vi "Global System.vi"() -> ()   [LabVIEW 2017]
uses:
  <vilib>/userdefined/High Color/IMAQdx.ctl
  <vilib>/vision/Pattern Matching.llb/IMAQ Curve Parameters.ctl
  <vilib>/vision/Image Controls.llb/IMAQ Image.ctl
  <vilib>/vision/Measure.llb/Edge Options.ctl
  <vilib>/vision/Measure.llb/Edge Polarity.ctl
  <vilib>/vision/Measure.llb/Straight Edge Options.ctl
  <vilib>/vision/Measure.llb/Straight Edge Process.ctl
  <vilib>/vision/Pattern Matching.llb/IMAQ Match Range Setting.ctl
panel:
  out "码枪结果":bool
  out "CR-CCD1字符定位参数":T4={"Rectangle"={"Left"=0, "Top"=0, "Right"=0, "Bottom"=0, "Rotation"=0.0}, "Settings"={"Curve Parameters"={"Extraction Mode"=0, "Edge Threshold"=35, "Edge Filter Size"=1, "Min Length"=25, "Row Search Step Size"=15, "Col Search Step Size"=15, "Max Endpoint Gap"=10, "Closed"=FALSE, "Subpixel"=FALSE}, "Match Mode"={"Rotation"=TRUE, "Scale"=FALSE, "Occlusion"=TRUE, "Reserved 1"=FALSE, "Reserved 2"=FALSE, "Reserved 3"=FALSE}, "Range Settings"=[{"Match Constraints"=0, "Min"=-17.0, "Max"=17.0}, {"Match Constraints"=2, "Min"=0.0, "Max"=25.0}], "Number of Matches"=1, "Minimum Match Score"=400.0, "SubPixel Accuracy"=FALSE, "Adv. Geometric Match Options 2"=[{"Setup Data Item"=21, "Item Value"=0.0}, {"Setup Data Item"=22, "Item Value"=1.0}]}, "Template File Path"=path "F:/Inspect System -2/Source Code/Template Program/程序1/字符定位模板.png"} {"Settings"."Curve Parameters"."Extraction Mode" items=["Normal", "Uniform Regions"]; "Settings"."Curve Parameters"."Edge Filter Size" items=["Fine", "Normal", "Contour Tracing"]; "Settings"."Curve Parameters"."Max Endpoint Gap" min=0; "Settings"."Curve Parameters"."Col Search Step Size" min=1 max=255 step=1; "Settings"."Curve Parameters"."Row Search Step Size" min=1 max=255 step=1; "Settings"."Curve Parameters"."Min Length" min=0; "Settings"."Curve Parameters"."Edge Threshold" min=1 max=350 step=1; "Settings"."Range Settings"."Max" format="%.2f"; "Settings"."Range Settings"."Min" format="%.2f"; "Settings"."Range Settings"."Match Constraints" items=["Rotation Angle (degrees)", "Scale Factor (%)", "Occlusion (%)"]; "Settings"."Adv. Geometric Match Options 2"."Setup Data Item" items=["Curve Extraction Mode", "Curve Edge Threshold", "Curve Edge Filter Size", "Min Curve Length", "Curve Row Search Step Size", "Curve Col Search Step Size", "Curve Max Endpoint Gap", "Extract Closed Curves", "Enable Subpixel Curve Extraction", "Enable Correlation Score", "Enable Subpixel Accuracy", "Subpixel Iterations", "Subpixel Tolerance", "Initial Match List Length", "Enable Target Template Curve Score", "Min Match Separation Distance", "Min Match Separation Angle", "Min Match Separation Scale", "Max Match Overlap", "Enable Coarse Result", "Enable Calibration Support", "Enable Contrast Reversal", "Search Strategy", "Refinement Match Factor", "Subpixel Match Factor"]; "Rectangle"."Rotation" format="%.2f"; "Rectangle"."Left" scale=0.0..1024.0; "Rectangle"."Right" scale=0.0..1024.0}
  out "扫码次数计数":dbl
  out "CR位置范围设定":T5={"位置1"={"上限"=726.0, "下限"=686.0}, "位置2"={"上限"=874.0, "下限"=834.0}, "位置3"={"上限"=997.0, "下限"=957.0}, "位置4"={"上限"=1139.0, "下限"=1099.0}, "位置5"={"上限"=1283.0, "下限"=1243.0}, "位置6"={"上限"=1429.0, "下限"=1389.0}, "位置7"={"上限"=1576.0, "下限"=1536.0}, "位置8"={"上限"=1728.0, "下限"=1688.0}, "位置9"={"上限"=1879.0, "下限"=1839.0}, "位置10"={"上限"=2036.0, "下限"=1996.0}}
  out "CR- 字符检测参数 2":T6={"Parameters (OCR/OCV 1)"={"Threshold Data"={"Method"=enum."Local", "Looking for"=1, "Color Mode"=0, "Kernel Size"={"Width"=32, "Height"=32}, "Ranges"=[{"Min"=1, "Max"=255}]}, "Reject Border"=TRUE, "Number Of Erosions"=0, "Size & Spacing"={"Segment Algorithm"=0, "Min Bounding Rect Width"=1, "Max Bounding Rect Width"=65536, "Min Bounding Rect Height"=1, "Max Bounding Rect Height"=65536, "Min Character Size"=20, "Max Character Size"=65536, "Min Char Spacing"=1, "Max Horiz Element Spacing"=1, "Max Vert Element Spacing"=0, "Max Space Distance"=65536}, "Read Options"={"Read Strategy"=1, "Read Resolution"=2, "Scale Dependant"=FALSE, "Aspect Ratio"=400, "Acceptance Level"=700, "Substitution Character"="?", "MultiLine"=TRUE}, "Valid Characters"=[], "Use Text Pattern"=FALSE, "Orientation"=0, "# Lines Expected"=0, "Number of Blocks"=4}, "Rectangle"={"Left"=0, "Top"=0, "Right"=0, "Bottom"=0, "Rotation"=0.0}, "字符长度判定"=0.0, "Reference System"={"Origin"={"X"=1245.2058, "Y"=1038.7815}, "Angle (deg)"=0.021420227, "Axis Reference"=0}, "File Path (字符库)"=path "D:/Inspect System/Source Code/Template Program/字符模板.abc", "File Path (连接件模板)"=path "D:/Inspect System/Source Code/Template Program/字符检测定位模板.png", "Url"="http://10.6.1.31:8080/MesInnerpackLineIO.asmx", "accessKey"="a45b2d3334ffs_\na45b2d3334ffs_"} {"Reference System"."Axis Reference" items=["Direct", "Indirect"]; "Rectangle"."Rotation" min=-90.0 max=90.0 step=1.0 format="%.2f"; "Rectangle"."Left" scale=0.0..1024.0; "Rectangle"."Right" scale=0.0..1024.0; "Parameters (OCR/OCV 1)"."Threshold Data"."Looking for" items=["Light on Dark", "Dark on Light"]; "Parameters (OCR/OCV 1)"."Threshold Data"."Color Mode" items=["RGB", "HSL", "HSV", "HSI"]; "Parameters (OCR/OCV 1)"."Size & Spacing"."Segment Algorithm" items=["None", "Shortest Segment", "Legacy Auto Split"]; "Parameters (OCR/OCV 1)"."Read Options"."Read Strategy" items=["Aggressive", "Conservative"]; "Parameters (OCR/OCV 1)"."Read Options"."Read Resolution" items=["Low", "Medium", "High"]; "Parameters (OCR/OCV 1)"."Valid Characters"."Pre-defined characters" items=["Any Character", "User-defined Characters", "Alphabetic", "Alphanumeric", "Uppercase Letters", "Lowercase Letters", "Decimal Digits", "Hexadecimal Digits", "Pattern", "Force Space"]; "Parameters (OCR/OCV 1)"."Orientation" items=["Baseline inside", "Baseline outside"]}
  in  "CR- 衬丝检测ROI参数":T8 {"Line 2"."Start X" scale=0.0..1024.0; "Line 2"."End X" scale=0.0..1024.0; "clamp Rectangle"."Rotation" min=-90.0 max=90.0 step=1.0 format="%.2f"; "clamp Rectangle"."Left" scale=0.0..1024.0; "clamp Rectangle"."Right" scale=0.0..1024.0; "Line 1"."Start X" scale=0.0..1024.0; "Line 1"."End X" scale=0.0..1024.0; "find straight edge Rectangle"."Rotation" min=-90.0 max=90.0 step=1.0 format="%.2f"; "find straight edge Rectangle"."Left" scale=0.0..1024.0; "find straight edge Rectangle"."Right" scale=0.0..1024.0}
  in  "衬丝检测基础参数":T9={"IsNorImage"=TRUE, "Exposure Values"=100289, "ImagePath"=path "C:/Users/hedongpo/Desktop/514-hdp/Alignment Assemble System/Test Picture/B/3.bmp"} caption="参数界面" {"Exposure Values" scale=0.0..200000.0}
  out "CR- 衬丝检测参数":T12={"Settings (Clamp (Rake) 1)"={"Contrast"=154, "Filter width"=4, "Steepness"=2, "Subsampling Ratio"=5, "Show Search Area"=TRUE, "Show Search Lines"=TRUE, "Show Edges Found"=TRUE, "Show Result"=TRUE}, "Options (Find Straight Edge 1)"={"Search Direction"=0, "Edge Options"={"Edge Polarity"=0, "Kernel Size"=3, "Width"=1, "Minimum Edge Strength"=65.0, "Interpolation Type"=enum."Bilinear Fixed", "Data Processing Method"=enum."Average"}, "Show Search Area"=TRUE, "Show Search Lines"=TRUE, "Show Edges Found"=TRUE, "Show Result"=TRUE, "Search Area Color"=65280, "Search Lines Color"=255, "Edge Locations Color"=16776960, "Result Color"=16711680, "Overlay Group Name"=""}, "相对距离设定"={"上限"=0.0, "下限"=0.0}, "衬丝直径设定"={"上限"=0.0, "下限"=0.0}, "保护套直径设定"={"上限"=0.0, "下限"=0.0}, "Edge Options (Edge Detector 1)"={"Edge Polarity"=0, "Kernel Size"=3, "Width"=3, "Minimum Edge Strength"=10.0, "Interpolation Type"=enum."Bilinear Fixed", "Data Processing Method"=enum."Average"}, "保护套标准位置"={"Start X"=0, "Start Y"=0, "End X"=0, "End Y"=0}} {"保护套标准位置"."Start X" scale=0.0..1024.0; "保护套标准位置"."End X" scale=0.0..1024.0; "Edge Options (Edge Detector 1)"."Edge Polarity" items=["All Edges", "Rising Edges", "Falling Edges"]; "Options (Find Straight Edge 1)"."Search Direction" items=["Left to Right", "Right to Left", "Top to Bottom", "Bottom to Top"]; "Options (Find Straight Edge 1)"."Edge Options"."Edge Polarity" items=["All Edges", "Rising Edges", "Falling Edges"]; "Options (Find Straight Edge 1)"."Edge Options"."Minimum Edge Strength" format="%.2f"; "Options (Find Straight Edge 1)"."Edge Options"."Width" step=2; "Options (Find Straight Edge 1)"."Edge Options"."Kernel Size" step=2}
  out "颗粒物检测1基础参数 2":T14={"IsNorImage"=TRUE, "Exposure Values"=100289, "ImagePath"=path "C:/Users/hedongpo/Desktop/514-hdp/Alignment Assemble System/Test Picture/B/3.bmp", "相机选择"="cam4"} caption="参数界面" {"Exposure Values" scale=0.0..200000.0}
  in  "字符检测基础参数":T9={"IsNorImage"=TRUE, "Exposure Values"=100289, "ImagePath"=path "C:/Users/hedongpo/Desktop/514-hdp/Alignment Assemble System/Test Picture/B/3.bmp"} caption="参数界面" {"Exposure Values" scale=0.0..200000.0}
  in  "扫码枪基础参数":T15 caption="参数界面"
  in  "CR导丝纤维毛发检测3参数":T16={"Curve Extraction Settings "={"Extraction Mode"=0, "Edge Threshold"=25, "Edge Filter Size"=1, "Min Length"=19, "Row Search Step Size"=5, "Col Search Step Size"=5, "Max Endpoint Gap"=10, "Closed"=FALSE, "Subpixel"=FALSE}, "Color Mode (Histogram 1)"=0, "Range (Threshold 1)"={"Lower value"=62.0, "Upper value"=255.0}, "Clamp Settings (Max Clamp 1)"={"Angle Range (+/-)"=10.0, "Edge Polarity"={"Start"=0, "End"=0}}, "Settings (Clamp (Rake) 1)"={"Contrast"=6, "Filter width"=5, "Steepness"=2, "Subsampling Ratio"=5, "Show Search Area"=TRUE, "Show Search Lines"=TRUE, "Show Edges Found"=TRUE, "Show Result"=TRUE}, "直径设定"={"Lower value"=62.0, "Upper value"=255.0}} {"Clamp Settings (Max Clamp 1)"."Edge Polarity"."Start" items=["Any", "Rising", "Falling"]; "Clamp Settings (Max Clamp 1)"."Edge Polarity"."End" items=["Any", "Rising", "Falling"]; "Color Mode (Histogram 1)" items=["RGB", "HSL", "HSV", "HSI"]; "Curve Extraction Settings"."Extraction Mode" items=["Normal", "Uniform Regions"]; "Curve Extraction Settings"."Edge Filter Size" items=["Fine", "Normal", "Contour Tracing"]; "Curve Extraction Settings"."Max Endpoint Gap" min=0; "Curve Extraction Settings"."Col Search Step Size" min=1 max=255 step=1; "Curve Extraction Settings"."Row Search Step Size" min=1 max=255 step=1; "Curve Extraction Settings"."Min Length" min=0; "Curve Extraction Settings"."Edge Threshold" min=1 max=350 step=1}
  in  "CR颗粒物检测3参数":T17={"Rectangle"={"Left"=0, "Top"=0, "Right"=0, "Bottom"=0, "Rotation"=0.0}, "Threshold Limits (Threshold 1)"={"Lower value"=6.0, "Upper value"=245.0}, "Keep/Remove Particles "=FALSE, "Connectivity 4/8 (8) "=TRUE, "Selection Values (Particle Filter 1)"=[{"Measurement Parameter"=35, "Range Lower Value"=80.0, "Range Upper Value"=16332.0, "Range"=FALSE, "Measurement Type"=FALSE}], "Corner Options (Feature Detection 1)"={"Detector type"=enum."Harris Corner", "Kernel size"=7, "Min Corner Point Strength"=32.0}, "Pyramid level (Feature Detection 1)"=3, "Method "=2, "Look For"=0, "Method 2"=2, "ROI Descriptor (Clamp (Rake) 1)"={"Global Rectangle"=[162, 394, 420, 1807], "Contours"=[{"ID"=enum."External", "Type"=12, "Coordinates"=[162, 394, 420, 1807, 0]}]}} {"Method" items=["clustering", "entropy", "metric", "moments", "inter-class variance"]; "Look For" items=["Bright Objects", "Dark Objects"]; "Method 2" items=["clustering", "entropy", "metric", "moments", "inter-class variance"]; "ROI Descriptor (Clamp (Rake) 1)"."Contours"."Type" items=["No Selection", "Point", "Line", "Rectangle", "Oval", "Polygon", "Freehand Region", "Annulus", "Unused2", "Unused3", "Broken Line", "Freehand Line", "Rotated Rectangle"]; "Selection Values (Particle Filter 1)"."Measurement Parameter" items=["Center of Mass X", "Center of Mass Y", "First Pixel X", "First Pixel Y", "Bounding Rect Left", "Bounding Rect Top", "Bounding Rect Right", "Bounding Rect Bottom", "Max Feret Diameter Start X", "Max Feret Diameter Start Y", "Max Feret Diameter End X", "Max Feret Diameter End Y", "Max Horiz. Segment Length Left", "Max Horiz. Segment Length Right", "Max Horiz. Segment Length Row", "-", "Bounding Rect Width", "Bounding Rect Height", "Bounding Rect Diagonal", "Perimeter", "Convex Hull Perimeter", "Holes' Perimeter", "Max Feret Diameter", "Equivalent Ellipse Major Axis", "Equivalent Ellipse Minor Axis", "Equivalent Ellipse Minor Axis (Feret)", "Equivalent Rect Long Side", "Equivalent Rect Short Side", "Equivalent Rect Diagonal", "Equivalent Rect Short Side (Feret)", "Average Horiz. Segment Length", "Average Vert. Segment Length", "Hydraulic Radius", "Waddel Disk Diameter", "-", "Area", "Holes' Area", "Particle & Holes' Area", "Convex Hull Area", "Image Area", "-", "Number of Holes", "Number of Horiz. Segments", "Number of Vert. Segments", "-", "Orientation", "Max Feret Diameter Orientation", "-", "% Area/Image Area", "% Area/(Particle & Holes' Area)", "Ratio of Equivalent Ellipse Axes", "Ratio of Equivalent Rect Sides", "-", "Elongation Factor", "Compactness Factor", "Heywood Circularity Factor", "Type Factor", "-", "Sum X", "Sum Y", "Sum XX", "Sum XY", "Sum YY", "Sum XXX", "Sum XXY", "Sum XYY", "Sum YYY", "-", "Moment of Inertia XX", "Moment of Inertia XY", "Moment of Inertia YY", "Moment of Inertia XXX", "Moment of Inertia XXY", "Moment of Inertia XYY", "Moment of Inertia YYY", "Norm. Moment of Inertia XX", "Norm. Moment of Inertia XY", "Norm. Moment of Inertia YY", "Norm. Moment of Inertia XXX", "Norm. Moment of Inertia XXY", "Norm. Moment of Inertia XYY", "Norm. Moment of Inertia YYY", "Hu Moment 1", "Hu Moment 2", "Hu Moment 3", "Hu Moment 4", "Hu Moment 5", "Hu Moment 6", "Hu Moment 7"]; "Rectangle"."Rotation" min=-90.0 max=90.0 step=1.0 format="%.2f"; "Rectangle"."Left" scale=0.0..1024.0; "Rectangle"."Right" scale=0.0..1024.0}
  in  "CR颗粒物检测2参数":T17={"Rectangle"={"Left"=0, "Top"=0, "Right"=0, "Bottom"=0, "Rotation"=0.0}, "Threshold Limits (Threshold 1)"={"Lower value"=6.0, "Upper value"=245.0}, "Keep/Remove Particles "=FALSE, "Connectivity 4/8 (8) "=TRUE, "Selection Values (Particle Filter 1)"=[{"Measurement Parameter"=35, "Range Lower Value"=80.0, "Range Upper Value"=16332.0, "Range"=FALSE, "Measurement Type"=FALSE}], "Corner Options (Feature Detection 1)"={"Detector type"=enum."Harris Corner", "Kernel size"=7, "Min Corner Point Strength"=32.0}, "Pyramid level (Feature Detection 1)"=3, "Method "=2, "Look For"=0, "Method 2"=2, "ROI Descriptor (Clamp (Rake) 1)"={"Global Rectangle"=[162, 394, 420, 1807], "Contours"=[{"ID"=enum."External", "Type"=12, "Coordinates"=[162, 394, 420, 1807, 0]}]}} {"Method" items=["clustering", "entropy", "metric", "moments", "inter-class variance"]; "Look For" items=["Bright Objects", "Dark Objects"]; "Method 2" items=["clustering", "entropy", "metric", "moments", "inter-class variance"]; "ROI Descriptor (Clamp (Rake) 1)"."Contours"."Type" items=["No Selection", "Point", "Line", "Rectangle", "Oval", "Polygon", "Freehand Region", "Annulus", "Unused2", "Unused3", "Broken Line", "Freehand Line", "Rotated Rectangle"]; "Selection Values (Particle Filter 1)"."Measurement Parameter" items=["Center of Mass X", "Center of Mass Y", "First Pixel X", "First Pixel Y", "Bounding Rect Left", "Bounding Rect Top", "Bounding Rect Right", "Bounding Rect Bottom", "Max Feret Diameter Start X", "Max Feret Diameter Start Y", "Max Feret Diameter End X", "Max Feret Diameter End Y", "Max Horiz. Segment Length Left", "Max Horiz. Segment Length Right", "Max Horiz. Segment Length Row", "-", "Bounding Rect Width", "Bounding Rect Height", "Bounding Rect Diagonal", "Perimeter", "Convex Hull Perimeter", "Holes' Perimeter", "Max Feret Diameter", "Equivalent Ellipse Major Axis", "Equivalent Ellipse Minor Axis", "Equivalent Ellipse Minor Axis (Feret)", "Equivalent Rect Long Side", "Equivalent Rect Short Side", "Equivalent Rect Diagonal", "Equivalent Rect Short Side (Feret)", "Average Horiz. Segment Length", "Average Vert. Segment Length", "Hydraulic Radius", "Waddel Disk Diameter", "-", "Area", "Holes' Area", "Particle & Holes' Area", "Convex Hull Area", "Image Area", "-", "Number of Holes", "Number of Horiz. Segments", "Number of Vert. Segments", "-", "Orientation", "Max Feret Diameter Orientation", "-", "% Area/Image Area", "% Area/(Particle & Holes' Area)", "Ratio of Equivalent Ellipse Axes", "Ratio of Equivalent Rect Sides", "-", "Elongation Factor", "Compactness Factor", "Heywood Circularity Factor", "Type Factor", "-", "Sum X", "Sum Y", "Sum XX", "Sum XY", "Sum YY", "Sum XXX", "Sum XXY", "Sum XYY", "Sum YYY", "-", "Moment of Inertia XX", "Moment of Inertia XY", "Moment of Inertia YY", "Moment of Inertia XXX", "Moment of Inertia XXY", "Moment of Inertia XYY", "Moment of Inertia YYY", "Norm. Moment of Inertia XX", "Norm. Moment of Inertia XY", "Norm. Moment of Inertia YY", "Norm. Moment of Inertia XXX", "Norm. Moment of Inertia XXY", "Norm. Moment of Inertia XYY", "Norm. Moment of Inertia YYY", "Hu Moment 1", "Hu Moment 2", "Hu Moment 3", "Hu Moment 4", "Hu Moment 5", "Hu Moment 6", "Hu Moment 7"]; "Rectangle"."Rotation" min=-90.0 max=90.0 step=1.0 format="%.2f"; "Rectangle"."Left" scale=0.0..1024.0; "Rectangle"."Right" scale=0.0..1024.0}
  in  "扫码枪参数":T18={"IsNorImage"=TRUE, "Exposure Values"=100289, "ImagePath"=path "C:/Users/hedongpo/Desktop/514-hdp/Alignment Assemble System/Test Picture/B/3.bmp", "数据输出"="", "结果显示"=FALSE} caption="参数界面" {"Exposure Values" scale=0.0..200000.0}
  in  "CR纤维毛发检测1参数":T16={"Curve Extraction Settings "={"Extraction Mode"=0, "Edge Threshold"=25, "Edge Filter Size"=1, "Min Length"=19, "Row Search Step Size"=5, "Col Search Step Size"=5, "Max Endpoint Gap"=10, "Closed"=FALSE, "Subpixel"=FALSE}, "Color Mode (Histogram 1)"=0, "Range (Threshold 1)"={"Lower value"=62.0, "Upper value"=255.0}, "Clamp Settings (Max Clamp 1)"={"Angle Range (+/-)"=10.0, "Edge Polarity"={"Start"=0, "End"=0}}, "Settings (Clamp (Rake) 1)"={"Contrast"=6, "Filter width"=5, "Steepness"=2, "Subsampling Ratio"=5, "Show Search Area"=TRUE, "Show Search Lines"=TRUE, "Show Edges Found"=TRUE, "Show Result"=TRUE}, "直径设定"={"Lower value"=62.0, "Upper value"=255.0}} {"Clamp Settings (Max Clamp 1)"."Edge Polarity"."Start" items=["Any", "Rising", "Falling"]; "Clamp Settings (Max Clamp 1)"."Edge Polarity"."End" items=["Any", "Rising", "Falling"]; "Color Mode (Histogram 1)" items=["RGB", "HSL", "HSV", "HSI"]; "Curve Extraction Settings"."Extraction Mode" items=["Normal", "Uniform Regions"]; "Curve Extraction Settings"."Edge Filter Size" items=["Fine", "Normal", "Contour Tracing"]; "Curve Extraction Settings"."Max Endpoint Gap" min=0; "Curve Extraction Settings"."Col Search Step Size" min=1 max=255 step=1; "Curve Extraction Settings"."Row Search Step Size" min=1 max=255 step=1; "Curve Extraction Settings"."Min Length" min=0; "Curve Extraction Settings"."Edge Threshold" min=1 max=350 step=1}
  out "CR纤维毛发检测1基础参数":T14={"IsNorImage"=TRUE, "Exposure Values"=100289, "ImagePath"=path "C:/Users/hedongpo/Desktop/514-hdp/Alignment Assemble System/Test Picture/B/3.bmp", "相机选择"="cam4"} caption="参数界面" {"Exposure Values" scale=0.0..200000.0}
  out "UI电源尾反面漏线参数":T19={"Rectangle"={"Left"=0, "Top"=0, "Right"=0, "Bottom"=0, "Rotation"=0.0}, "模板路径"=path "C:/Users/delluser001/Desktop/PowerLine Inspect System/Source Code/Template Program/potteryTemplete/Color.png", "Match Mode "=0, "Minimum Match Score "=800.0, "Number of Matches Requested"=1, "Rotation Angle Ranges (degrees)"=[{"Min"=-180.0, "Max"=180.0}], "Color Sensitivity "=0, "Match Offset"={"X"=0.0, "Y"=0.0}, "Color Score Weight "=500.0, "Search Strategy "=0, "Subpixel Accuracy "=FALSE, "Range (Threshold 1)"={"Lower value"=148.0, "Upper value"=255.0}} {"Rectangle"."Rotation" format="%.2f"; "Rectangle"."Left" scale=0.0..1024.0; "Rectangle"."Right" scale=0.0..1024.0; "Search Strategy" items=["Conservative", "Balance", "Aggressive", "Very Aggressive"]; "Color Sensitivity" items=["Low Sensitivity", "Medium Sensitivity", "High Sensitivity"]; "Match Mode" items=["Shift Invariant", "Rotation Invariant"]}
  out "UI电源尾反面漏线基础参数":T9={"IsNorImage"=TRUE, "Exposure Values"=100289, "ImagePath"=path "C:/Users/hedongpo/Desktop/514-hdp/Alignment Assemble System/Test Picture/B/3.bmp"} caption="参数界面" {"Exposure Values" scale=0.0..200000.0}
  out "UI电源尾反面标签2参数":T20={"Rectangle"={"Left"=0, "Top"=0, "Right"=0, "Bottom"=0, "Rotation"=0.0}, "Algorithm "=2, "Parameters"={"Number of Matches Requested"=1, "Minimum Match Score"=800.0, "Angle Ranges"=[{"Start Angle"=-180.0, "End Angle"=180.0}]}, "Advanced Options "=[{"Item"=102, "Value"=10.0}, {"Item"=106, "Value"=300.0}, {"Item"=107, "Value"=0.0}, {"Item"=108, "Value"=6.0}, {"Item"=109, "Value"=1.0}, {"Item"=114, "Value"=25.0}, {"Item"=111, "Value"=20.0}, {"Item"=112, "Value"=10.0}, {"Item"=113, "Value"=20.0}, {"Item"=103, "Value"=1.0}, {"Item"=104, "Value"=20.0}, {"Item"=105, "Value"=0.0}, {"Item"=100, "Value"=5.0}], "模板路径"=path "", "Color Plane "=0} {"Color Plane" items=["Red", "Green", "Blue", "Hue", "Saturation", "Luminance", "Value", "Intensity"]; "Advanced Options"."Item" items=["LD Sampling - Minimum Constrast"=0, "LD Sampling - Enable Subpixel Accuracy"=1, "LD Sampling - Search Strategy"=2, "LD Sampling - Subpixel Iterations"=3, "LD Sampling - Subpixel Tolerance"=4, "LD Sampling - Initial Match List Length"=5, "LD Sampling - Match List Reduction Factor"=6, "LD Sampling - Initial Step Size"=7, "LD Sampling - Intermediate Angular Accuracy"=8, "-"=9, "Pyramid - Max Pyramid Level"=100, "Pyramid - Minimum Contrast"=102, "Pyramid - Enable Subpixel Accuracy"=103, "Pyramid - Subpixel Iterations"=104, "Pyramid - Subpixel Tolerance"=105, "Pyramid - Initial Match List Length"=106, "Pyramid - Match List Reduction Factor"=107, "Pyramid - Intermediate Angular Accuracy"=108, "Pyramid - Process Border Matches"=109, "Pyramid - Min Match Separation Distance"=111, "Pyramid - Min Match Separation Angle"=112, "Pyramid - Max Match Overlap"=113, "Pyramid - Max Cache in MB"=114, "Pyramid - Clear Cache"=115, "-"=116, "Enable Defect Map"=200]; "Algorithm" items=["All", "Low Discrepancy Sampling", "Grayscale Value Pyramid", "Gradients Pyramid"]; "Rectangle"."Rotation" format="%.2f"; "Rectangle"."Left" scale=0.0..1024.0; "Rectangle"."Right" scale=0.0..1024.0}
  out "UI电源尾反面标签2基础参数":T9={"IsNorImage"=TRUE, "Exposure Values"=100289, "ImagePath"=path "C:/Users/hedongpo/Desktop/514-hdp/Alignment Assemble System/Test Picture/B/3.bmp"} caption="参数界面" {"Exposure Values" scale=0.0..200000.0}
  out "UI电源尾反面标签1参数":T20={"Rectangle"={"Left"=0, "Top"=0, "Right"=0, "Bottom"=0, "Rotation"=0.0}, "Algorithm "=2, "Parameters"={"Number of Matches Requested"=1, "Minimum Match Score"=800.0, "Angle Ranges"=[{"Start Angle"=-180.0, "End Angle"=180.0}]}, "Advanced Options "=[{"Item"=102, "Value"=10.0}, {"Item"=106, "Value"=300.0}, {"Item"=107, "Value"=0.0}, {"Item"=108, "Value"=6.0}, {"Item"=109, "Value"=1.0}, {"Item"=114, "Value"=25.0}, {"Item"=111, "Value"=20.0}, {"Item"=112, "Value"=10.0}, {"Item"=113, "Value"=20.0}, {"Item"=103, "Value"=1.0}, {"Item"=104, "Value"=20.0}, {"Item"=105, "Value"=0.0}, {"Item"=100, "Value"=5.0}], "模板路径"=path "", "Color Plane "=0} {"Color Plane" items=["Red", "Green", "Blue", "Hue", "Saturation", "Luminance", "Value", "Intensity"]; "Advanced Options"."Item" items=["LD Sampling - Minimum Constrast"=0, "LD Sampling - Enable Subpixel Accuracy"=1, "LD Sampling - Search Strategy"=2, "LD Sampling - Subpixel Iterations"=3, "LD Sampling - Subpixel Tolerance"=4, "LD Sampling - Initial Match List Length"=5, "LD Sampling - Match List Reduction Factor"=6, "LD Sampling - Initial Step Size"=7, "LD Sampling - Intermediate Angular Accuracy"=8, "-"=9, "Pyramid - Max Pyramid Level"=100, "Pyramid - Minimum Contrast"=102, "Pyramid - Enable Subpixel Accuracy"=103, "Pyramid - Subpixel Iterations"=104, "Pyramid - Subpixel Tolerance"=105, "Pyramid - Initial Match List Length"=106, "Pyramid - Match List Reduction Factor"=107, "Pyramid - Intermediate Angular Accuracy"=108, "Pyramid - Process Border Matches"=109, "Pyramid - Min Match Separation Distance"=111, "Pyramid - Min Match Separation Angle"=112, "Pyramid - Max Match Overlap"=113, "Pyramid - Max Cache in MB"=114, "Pyramid - Clear Cache"=115, "-"=116, "Enable Defect Map"=200]; "Algorithm" items=["All", "Low Discrepancy Sampling", "Grayscale Value Pyramid", "Gradients Pyramid"]; "Rectangle"."Rotation" format="%.2f"; "Rectangle"."Left" scale=0.0..1024.0; "Rectangle"."Right" scale=0.0..1024.0}
  out "UI电源尾反面标签1基础参数":T9={"IsNorImage"=TRUE, "Exposure Values"=100289, "ImagePath"=path "C:/Users/hedongpo/Desktop/514-hdp/Alignment Assemble System/Test Picture/B/3.bmp"} caption="参数界面" {"Exposure Values" scale=0.0..200000.0}
  out "UI电源尾正面漏线参数":T19={"Rectangle"={"Left"=0, "Top"=0, "Right"=0, "Bottom"=0, "Rotation"=0.0}, "模板路径"=path "C:/Users/delluser001/Desktop/PowerLine Inspect System/Source Code/Template Program/potteryTemplete/Color.png", "Match Mode "=0, "Minimum Match Score "=800.0, "Number of Matches Requested"=1, "Rotation Angle Ranges (degrees)"=[{"Min"=-180.0, "Max"=180.0}], "Color Sensitivity "=0, "Match Offset"={"X"=0.0, "Y"=0.0}, "Color Score Weight "=500.0, "Search Strategy "=0, "Subpixel Accuracy "=FALSE, "Range (Threshold 1)"={"Lower value"=177.0, "Upper value"=255.0}} {"Rectangle"."Rotation" format="%.2f"; "Rectangle"."Left" scale=0.0..1024.0; "Rectangle"."Right" scale=0.0..1024.0; "Search Strategy" items=["Conservative", "Balance", "Aggressive", "Very Aggressive"]; "Color Sensitivity" items=["Low Sensitivity", "Medium Sensitivity", "High Sensitivity"]; "Match Mode" items=["Shift Invariant", "Rotation Invariant"]}
  out "UI电源尾正面漏线基础参数":T9={"IsNorImage"=TRUE, "Exposure Values"=100289, "ImagePath"=path "C:/Users/hedongpo/Desktop/514-hdp/Alignment Assemble System/Test Picture/B/3.bmp"} caption="参数界面" {"Exposure Values" scale=0.0..200000.0}
  out "CR导丝缺损检测3参数":T20={"Rectangle"={"Left"=0, "Top"=0, "Right"=0, "Bottom"=0, "Rotation"=0.0}, "Algorithm "=2, "Parameters"={"Number of Matches Requested"=1, "Minimum Match Score"=800.0, "Angle Ranges"=[{"Start Angle"=-180.0, "End Angle"=180.0}]}, "Advanced Options "=[{"Item"=102, "Value"=10.0}, {"Item"=106, "Value"=300.0}, {"Item"=107, "Value"=0.0}, {"Item"=108, "Value"=6.0}, {"Item"=109, "Value"=1.0}, {"Item"=114, "Value"=25.0}, {"Item"=111, "Value"=20.0}, {"Item"=112, "Value"=10.0}, {"Item"=113, "Value"=20.0}, {"Item"=103, "Value"=1.0}, {"Item"=104, "Value"=20.0}, {"Item"=105, "Value"=0.0}, {"Item"=100, "Value"=5.0}], "模板路径"=path "", "Color Plane "=0} {"Color Plane" items=["Red", "Green", "Blue", "Hue", "Saturation", "Luminance", "Value", "Intensity"]; "Advanced Options"."Item" items=["LD Sampling - Minimum Constrast"=0, "LD Sampling - Enable Subpixel Accuracy"=1, "LD Sampling - Search Strategy"=2, "LD Sampling - Subpixel Iterations"=3, "LD Sampling - Subpixel Tolerance"=4, "LD Sampling - Initial Match List Length"=5, "LD Sampling - Match List Reduction Factor"=6, "LD Sampling - Initial Step Size"=7, "LD Sampling - Intermediate Angular Accuracy"=8, "-"=9, "Pyramid - Max Pyramid Level"=100, "Pyramid - Minimum Contrast"=102, "Pyramid - Enable Subpixel Accuracy"=103, "Pyramid - Subpixel Iterations"=104, "Pyramid - Subpixel Tolerance"=105, "Pyramid - Initial Match List Length"=106, "Pyramid - Match List Reduction Factor"=107, "Pyramid - Intermediate Angular Accuracy"=108, "Pyramid - Process Border Matches"=109, "Pyramid - Min Match Separation Distance"=111, "Pyramid - Min Match Separation Angle"=112, "Pyramid - Max Match Overlap"=113, "Pyramid - Max Cache in MB"=114, "Pyramid - Clear Cache"=115, "-"=116, "Enable Defect Map"=200]; "Algorithm" items=["All", "Low Discrepancy Sampling", "Grayscale Value Pyramid", "Gradients Pyramid"]; "Rectangle"."Rotation" format="%.2f"; "Rectangle"."Left" scale=0.0..1024.0; "Rectangle"."Right" scale=0.0..1024.0}
  out "UI电源线尾正面标签2基础参数":T9={"IsNorImage"=TRUE, "Exposure Values"=100289, "ImagePath"=path "C:/Users/hedongpo/Desktop/514-hdp/Alignment Assemble System/Test Picture/B/3.bmp"} caption="参数界面" {"Exposure Values" scale=0.0..200000.0}
  out "UI电源线尾正面标签1参数":T20={"Rectangle"={"Left"=0, "Top"=0, "Right"=0, "Bottom"=0, "Rotation"=0.0}, "Algorithm "=2, "Parameters"={"Number of Matches Requested"=1, "Minimum Match Score"=800.0, "Angle Ranges"=[{"Start Angle"=-180.0, "End Angle"=180.0}]}, "Advanced Options "=[{"Item"=102, "Value"=10.0}, {"Item"=106, "Value"=300.0}, {"Item"=107, "Value"=0.0}, {"Item"=108, "Value"=6.0}, {"Item"=109, "Value"=1.0}, {"Item"=114, "Value"=25.0}, {"Item"=111, "Value"=20.0}, {"Item"=112, "Value"=10.0}, {"Item"=113, "Value"=20.0}, {"Item"=103, "Value"=1.0}, {"Item"=104, "Value"=20.0}, {"Item"=105, "Value"=0.0}, {"Item"=100, "Value"=5.0}], "模板路径"=path "", "Color Plane "=0} {"Color Plane" items=["Red", "Green", "Blue", "Hue", "Saturation", "Luminance", "Value", "Intensity"]; "Advanced Options"."Item" items=["LD Sampling - Minimum Constrast"=0, "LD Sampling - Enable Subpixel Accuracy"=1, "LD Sampling - Search Strategy"=2, "LD Sampling - Subpixel Iterations"=3, "LD Sampling - Subpixel Tolerance"=4, "LD Sampling - Initial Match List Length"=5, "LD Sampling - Match List Reduction Factor"=6, "LD Sampling - Initial Step Size"=7, "LD Sampling - Intermediate Angular Accuracy"=8, "-"=9, "Pyramid - Max Pyramid Level"=100, "Pyramid - Minimum Contrast"=102, "Pyramid - Enable Subpixel Accuracy"=103, "Pyramid - Subpixel Iterations"=104, "Pyramid - Subpixel Tolerance"=105, "Pyramid - Initial Match List Length"=106, "Pyramid - Match List Reduction Factor"=107, "Pyramid - Intermediate Angular Accuracy"=108, "Pyramid - Process Border Matches"=109, "Pyramid - Min Match Separation Distance"=111, "Pyramid - Min Match Separation Angle"=112, "Pyramid - Max Match Overlap"=113, "Pyramid - Max Cache in MB"=114, "Pyramid - Clear Cache"=115, "-"=116, "Enable Defect Map"=200]; "Algorithm" items=["All", "Low Discrepancy Sampling", "Grayscale Value Pyramid", "Gradients Pyramid"]; "Rectangle"."Rotation" format="%.2f"; "Rectangle"."Left" scale=0.0..1024.0; "Rectangle"."Right" scale=0.0..1024.0}
  out "UI电源线尾正面标签1基础参数":T9={"IsNorImage"=TRUE, "Exposure Values"=100289, "ImagePath"=path "C:/Users/hedongpo/Desktop/514-hdp/Alignment Assemble System/Test Picture/B/3.bmp"} caption="参数界面" {"Exposure Values" scale=0.0..200000.0}
  out "CR导丝缺损检测3基础参数":T9={"IsNorImage"=TRUE, "Exposure Values"=100289, "ImagePath"=path "C:/Users/hedongpo/Desktop/514-hdp/Alignment Assemble System/Test Picture/B/3.bmp"} caption="参数界面" {"Exposure Values" scale=0.0..200000.0}
  out "CR导丝纤维毛发检测3基础参数":T9={"IsNorImage"=TRUE, "Exposure Values"=100289, "ImagePath"=path "C:/Users/hedongpo/Desktop/514-hdp/Alignment Assemble System/Test Picture/B/3.bmp"} caption="参数界面" {"Exposure Values" scale=0.0..200000.0}
  out "CR导丝颗粒物检测3基础参数":T9={"IsNorImage"=TRUE, "Exposure Values"=100289, "ImagePath"=path "C:/Users/hedongpo/Desktop/514-hdp/Alignment Assemble System/Test Picture/B/3.bmp"} caption="参数界面" {"Exposure Values" scale=0.0..200000.0}
  out "CR导丝划痕检测3参数":T20={"Rectangle"={"Left"=0, "Top"=0, "Right"=0, "Bottom"=0, "Rotation"=0.0}, "Algorithm "=2, "Parameters"={"Number of Matches Requested"=1, "Minimum Match Score"=800.0, "Angle Ranges"=[{"Start Angle"=-180.0, "End Angle"=180.0}]}, "Advanced Options "=[{"Item"=102, "Value"=10.0}, {"Item"=106, "Value"=300.0}, {"Item"=107, "Value"=0.0}, {"Item"=108, "Value"=6.0}, {"Item"=109, "Value"=1.0}, {"Item"=114, "Value"=25.0}, {"Item"=111, "Value"=20.0}, {"Item"=112, "Value"=10.0}, {"Item"=113, "Value"=20.0}, {"Item"=103, "Value"=1.0}, {"Item"=104, "Value"=20.0}, {"Item"=105, "Value"=0.0}, {"Item"=100, "Value"=5.0}], "模板路径"=path "", "Color Plane "=0} {"Color Plane" items=["Red", "Green", "Blue", "Hue", "Saturation", "Luminance", "Value", "Intensity"]; "Advanced Options"."Item" items=["LD Sampling - Minimum Constrast"=0, "LD Sampling - Enable Subpixel Accuracy"=1, "LD Sampling - Search Strategy"=2, "LD Sampling - Subpixel Iterations"=3, "LD Sampling - Subpixel Tolerance"=4, "LD Sampling - Initial Match List Length"=5, "LD Sampling - Match List Reduction Factor"=6, "LD Sampling - Initial Step Size"=7, "LD Sampling - Intermediate Angular Accuracy"=8, "-"=9, "Pyramid - Max Pyramid Level"=100, "Pyramid - Minimum Contrast"=102, "Pyramid - Enable Subpixel Accuracy"=103, "Pyramid - Subpixel Iterations"=104, "Pyramid - Subpixel Tolerance"=105, "Pyramid - Initial Match List Length"=106, "Pyramid - Match List Reduction Factor"=107, "Pyramid - Intermediate Angular Accuracy"=108, "Pyramid - Process Border Matches"=109, "Pyramid - Min Match Separation Distance"=111, "Pyramid - Min Match Separation Angle"=112, "Pyramid - Max Match Overlap"=113, "Pyramid - Max Cache in MB"=114, "Pyramid - Clear Cache"=115, "-"=116, "Enable Defect Map"=200]; "Algorithm" items=["All", "Low Discrepancy Sampling", "Grayscale Value Pyramid", "Gradients Pyramid"]; "Rectangle"."Rotation" format="%.2f"; "Rectangle"."Left" scale=0.0..1024.0; "Rectangle"."Right" scale=0.0..1024.0}
  out "CR导丝划痕检测3基础参数":T9={"IsNorImage"=TRUE, "Exposure Values"=100289, "ImagePath"=path "C:/Users/hedongpo/Desktop/514-hdp/Alignment Assemble System/Test Picture/B/3.bmp"} caption="参数界面" {"Exposure Values" scale=0.0..200000.0}
  out "CR导丝缺损检测2参数":T20={"Rectangle"={"Left"=0, "Top"=0, "Right"=0, "Bottom"=0, "Rotation"=0.0}, "Algorithm "=2, "Parameters"={"Number of Matches Requested"=1, "Minimum Match Score"=800.0, "Angle Ranges"=[{"Start Angle"=-180.0, "End Angle"=180.0}]}, "Advanced Options "=[{"Item"=102, "Value"=10.0}, {"Item"=106, "Value"=300.0}, {"Item"=107, "Value"=0.0}, {"Item"=108, "Value"=6.0}, {"Item"=109, "Value"=1.0}, {"Item"=114, "Value"=25.0}, {"Item"=111, "Value"=20.0}, {"Item"=112, "Value"=10.0}, {"Item"=113, "Value"=20.0}, {"Item"=103, "Value"=1.0}, {"Item"=104, "Value"=20.0}, {"Item"=105, "Value"=0.0}, {"Item"=100, "Value"=5.0}], "模板路径"=path "", "Color Plane "=0} {"Color Plane" items=["Red", "Green", "Blue", "Hue", "Saturation", "Luminance", "Value", "Intensity"]; "Advanced Options"."Item" items=["LD Sampling - Minimum Constrast"=0, "LD Sampling - Enable Subpixel Accuracy"=1, "LD Sampling - Search Strategy"=2, "LD Sampling - Subpixel Iterations"=3, "LD Sampling - Subpixel Tolerance"=4, "LD Sampling - Initial Match List Length"=5, "LD Sampling - Match List Reduction Factor"=6, "LD Sampling - Initial Step Size"=7, "LD Sampling - Intermediate Angular Accuracy"=8, "-"=9, "Pyramid - Max Pyramid Level"=100, "Pyramid - Minimum Contrast"=102, "Pyramid - Enable Subpixel Accuracy"=103, "Pyramid - Subpixel Iterations"=104, "Pyramid - Subpixel Tolerance"=105, "Pyramid - Initial Match List Length"=106, "Pyramid - Match List Reduction Factor"=107, "Pyramid - Intermediate Angular Accuracy"=108, "Pyramid - Process Border Matches"=109, "Pyramid - Min Match Separation Distance"=111, "Pyramid - Min Match Separation Angle"=112, "Pyramid - Max Match Overlap"=113, "Pyramid - Max Cache in MB"=114, "Pyramid - Clear Cache"=115, "-"=116, "Enable Defect Map"=200]; "Algorithm" items=["All", "Low Discrepancy Sampling", "Grayscale Value Pyramid", "Gradients Pyramid"]; "Rectangle"."Rotation" format="%.2f"; "Rectangle"."Left" scale=0.0..1024.0; "Rectangle"."Right" scale=0.0..1024.0}
  out "CR导丝缺损检测2基础参数":T9={"IsNorImage"=TRUE, "Exposure Values"=100289, "ImagePath"=path "C:/Users/hedongpo/Desktop/514-hdp/Alignment Assemble System/Test Picture/B/3.bmp"} caption="参数界面" {"Exposure Values" scale=0.0..200000.0}
  in  "CR导丝纤维毛发检测2参数":T21={"Max Number"=11.0, "Curve Extraction Settings "={"Extraction Mode"=0, "Edge Threshold"=25, "Edge Filter Size"=1, "Min Length"=19, "Row Search Step Size"=5, "Col Search Step Size"=5, "Max Endpoint Gap"=10, "Closed"=FALSE, "Subpixel"=FALSE}, "Color Mode (Histogram 1)"=0, "Range (Threshold 1)"={"Lower value"=62.0, "Upper value"=255.0}, "Clamp Settings (Max Clamp 1)"={"Angle Range (+/-)"=10.0, "Edge Polarity"={"Start"=0, "End"=0}}} {"Clamp Settings (Max Clamp 1)"."Edge Polarity"."Start" items=["Any", "Rising", "Falling"]; "Clamp Settings (Max Clamp 1)"."Edge Polarity"."End" items=["Any", "Rising", "Falling"]; "Color Mode (Histogram 1)" items=["RGB", "HSL", "HSV", "HSI"]; "Curve Extraction Settings"."Extraction Mode" items=["Normal", "Uniform Regions"]; "Curve Extraction Settings"."Edge Filter Size" items=["Fine", "Normal", "Contour Tracing"]; "Curve Extraction Settings"."Max Endpoint Gap" min=0; "Curve Extraction Settings"."Col Search Step Size" min=1 max=255 step=1; "Curve Extraction Settings"."Row Search Step Size" min=1 max=255 step=1; "Curve Extraction Settings"."Min Length" min=0; "Curve Extraction Settings"."Edge Threshold" min=1 max=350 step=1}
  out "CR导丝纤维毛发检测2基础参数":T9={"IsNorImage"=TRUE, "Exposure Values"=100289, "ImagePath"=path "C:/Users/hedongpo/Desktop/514-hdp/Alignment Assemble System/Test Picture/B/3.bmp"} caption="参数界面" {"Exposure Values" scale=0.0..200000.0}
  out "CR颗粒物检测2基础参数":T9={"IsNorImage"=TRUE, "Exposure Values"=100289, "ImagePath"=path "C:/Users/hedongpo/Desktop/514-hdp/Alignment Assemble System/Test Picture/B/3.bmp"} caption="参数界面" {"Exposure Values" scale=0.0..200000.0}
  in  "Global Variable":T22(tab)=enum."HW Run Status"
  out "ADODB._Connection Out":refnum<k7>
  out "CCD5":T23[](array[typedef])
  out "CCD4":T23[](array[typedef])
  out "CCD3":T23[](array[typedef])
  in  "Session Out CCD1":T13="cam1"
  out "表面检测判定":bool
  out "穿管检测判定":bool
  in  "Session Out CCD0":T13="cam0"
  in  "Session Out CCD5":T13="cam0"
  in  "Session Out CCD6":T13="cam6"
  in  "Session Out CCD4":T13="cam0"
  in  "FailNumber":string
  in  "PassNumber":string
  in  "Totalnumber":string
  in  "曝光值":i64=500 caption="ValueI64" min=500 max=5000000
  out "CCD2 Trigle Signal":bool
  in  "铜环拍照计数":i32
  in  "孔径拍照计数":i32
  out "Image":T23(plugin-control)
  out "CCD1 Trigle Signal":bool
  out "cam1":T13
  out "cam0":T13
  in  "Session Out CCD3":T13="cam0"
  in  "参数K":string
  in  "单位距离":string
  in  "参数B":string
  in  "校正像素值":string
  in  "TCP PLC Connect":refnum<k5>
  in  "Session Out CCD2":T13="cam0"
  in  "时间":dbl
  in  "相对角度值":dbl
  in  "相对中心Y值":dbl
  in  "相对中心X值":dbl
  out "A1 EXIT":bool
  out "产品型号选择 EXIT":bool
  out "PLC 连接":bool
  out "Paus":bool
  out "EMG":bool
  out "ref path":path
  in  "测试历史记录":string[][](table)=[["", ""]]
  out "exit app?":bool
  out "SWS":bool[](array[boolean])
  in  "sys error":errorcluster
  out "HWS":bool[](array[boolean])
  in  "emg rst Index":cluster{"emg":i32, "rst":i32, "active 0/1":i32}={"emg"=1, "rst"=4, "active 0/1"=0}
  out "queue":T24
  in  "DI Task":refnum<k21>
  in  "DO Task":refnum<k21>
  in  "AO Task":refnum<k21>
  in  "AI Task":refnum<k21>
  out "G_Status 2":bool
  out "自动触发计时器":bool
  out "G_Status 1":bool
  in  "test info E":string[](array[string])
  in  "test info C":string[](array[string])
  in  "Control caption C":string[](array[string])
  in  "Control caption E":string[](array[string])
  in  "Language code":string
  in  "test info index":i32
  in  "login user info":T25
  in  "User group availabe":bool[](array[boolean])
  in  "Login mode":bool[](array[boolean])
  in  "User group name":string[](array[string])
  in  "Domain":enum16{"Manager", "Engineer", "Operator"}(ring)
  out "CR导丝上料一致性参数":T28={"Rectangle"={"Left"=0, "Top"=0, "Right"=0, "Bottom"=0, "Rotation"=0.0}, "Find Straight Edge 1"={"Number of Lines"=1, "Type"=enum."First Edge Rake", "Min. Score"=10.0, "Max. Score"=1000.0, "Orientation"=0.0, "Angle Range"=45.0, "Angle Tolerance"=1.0, "Step Size"=11, "Min. SNR (db)"=0.0, "Min. Points (%)"=25.0, "Hough Iterations"=5}, "Process (Edge Detector 1)"=enum."Get All Edges", "Edge Options (Edge Detector 1)"={"Edge Polarity"=0, "Kernel Size"=9, "Width"=1, "Minimum Edge Strength"=8.0, "Interpolation Type"=enum."Bilinear Fixed", "Data Processing Method"=enum."Average"}, "Options (Find Straight Edge 1)"={"Search Direction"=0, "Edge Options"={"Edge Polarity"=0, "Kernel Size"=3, "Width"=1, "Minimum Edge Strength"=32.0, "Interpolation Type"=enum."Bilinear Fixed", "Data Processing Method"=enum."Average"}, "Show Search Area"=TRUE, "Show Search Lines"=TRUE, "Show Edges Found"=TRUE, "Show Result"=TRUE, "Search Area Color"=65280, "Search Lines Color"=255, "Edge Locations Color"=16776960, "Result Color"=16711680, "Overlay Group Name"=""}, "Parameters (Pattern Matching 1)"={"Number of Matches Requested"=1, "Minimum Match Score"=799.0, "Angle Ranges"=[{"Start Angle"=-180.0, "End Angle"=180.0}, {"Start Angle"=0.0, "End Angle"=360.0}]}, "Template File Path (Pattern Matching 1)"=path "D:/Inspect System/Source Code/Template Program/一致性模板.png"} {"Options (Find Straight Edge 1)"."Search Direction" items=["Left to Right", "Right to Left", "Top to Bottom", "Bottom to Top"]; "Options (Find Straight Edge 1)"."Edge Options"."Edge Polarity" items=["All Edges", "Rising Edges", "Falling Edges"]; "Options (Find Straight Edge 1)"."Edge Options"."Minimum Edge Strength" format="%.2f"; "Options (Find Straight Edge 1)"."Edge Options"."Width" step=2; "Options (Find Straight Edge 1)"."Edge Options"."Kernel Size" step=2; "Edge Options (Edge Detector 1)"."Edge Polarity" items=["All Edges", "Rising Edges", "Falling Edges"]; "Find Straight Edge 1"."Min. Points (%)" min=0.0 max=100.0; "Find Straight Edge 1"."Min. SNR (db)" min=0.0; "Find Straight Edge 1"."Max. Score" min=0.0 max=1024.0; "Find Straight Edge 1"."Min. Score" min=0.0 max=1024.0 step=1.0; "Rectangle"."Rotation" format="%.2f"; "Rectangle"."Left" scale=0.0..1024.0; "Rectangle"."Right" scale=0.0..1024.0}
  out "CR导丝上料一致性基础参数":T9={"IsNorImage"=TRUE, "Exposure Values"=100289, "ImagePath"=path "C:/Users/hedongpo/Desktop/514-hdp/Alignment Assemble System/Test Picture/B/3.bmp"} caption="参数界面" {"Exposure Values" scale=0.0..200000.0}
  out "导丝颗粒物检测1参数":T17={"Rectangle"={"Left"=0, "Top"=0, "Right"=0, "Bottom"=0, "Rotation"=0.0}, "Threshold Limits (Threshold 1)"={"Lower value"=6.0, "Upper value"=245.0}, "Keep/Remove Particles "=FALSE, "Connectivity 4/8 (8) "=TRUE, "Selection Values (Particle Filter 1)"=[{"Measurement Parameter"=35, "Range Lower Value"=80.0, "Range Upper Value"=16332.0, "Range"=FALSE, "Measurement Type"=FALSE}], "Corner Options (Feature Detection 1)"={"Detector type"=enum."Harris Corner", "Kernel size"=7, "Min Corner Point Strength"=32.0}, "Pyramid level (Feature Detection 1)"=3, "Method "=2, "Look For"=0, "Method 2"=2, "ROI Descriptor (Clamp (Rake) 1)"={"Global Rectangle"=[162, 394, 420, 1807], "Contours"=[{"ID"=enum."External", "Type"=12, "Coordinates"=[162, 394, 420, 1807, 0]}]}} {"Method" items=["clustering", "entropy", "metric", "moments", "inter-class variance"]; "Look For" items=["Bright Objects", "Dark Objects"]; "Method 2" items=["clustering", "entropy", "metric", "moments", "inter-class variance"]; "ROI Descriptor (Clamp (Rake) 1)"."Contours"."Type" items=["No Selection", "Point", "Line", "Rectangle", "Oval", "Polygon", "Freehand Region", "Annulus", "Unused2", "Unused3", "Broken Line", "Freehand Line", "Rotated Rectangle"]; "Selection Values (Particle Filter 1)"."Measurement Parameter" items=["Center of Mass X", "Center of Mass Y", "First Pixel X", "First Pixel Y", "Bounding Rect Left", "Bounding Rect Top", "Bounding Rect Right", "Bounding Rect Bottom", "Max Feret Diameter Start X", "Max Feret Diameter Start Y", "Max Feret Diameter End X", "Max Feret Diameter End Y", "Max Horiz. Segment Length Left", "Max Horiz. Segment Length Right", "Max Horiz. Segment Length Row", "-", "Bounding Rect Width", "Bounding Rect Height", "Bounding Rect Diagonal", "Perimeter", "Convex Hull Perimeter", "Holes' Perimeter", "Max Feret Diameter", "Equivalent Ellipse Major Axis", "Equivalent Ellipse Minor Axis", "Equivalent Ellipse Minor Axis (Feret)", "Equivalent Rect Long Side", "Equivalent Rect Short Side", "Equivalent Rect Diagonal", "Equivalent Rect Short Side (Feret)", "Average Horiz. Segment Length", "Average Vert. Segment Length", "Hydraulic Radius", "Waddel Disk Diameter", "-", "Area", "Holes' Area", "Particle & Holes' Area", "Convex Hull Area", "Image Area", "-", "Number of Holes", "Number of Horiz. Segments", "Number of Vert. Segments", "-", "Orientation", "Max Feret Diameter Orientation", "-", "% Area/Image Area", "% Area/(Particle & Holes' Area)", "Ratio of Equivalent Ellipse Axes", "Ratio of Equivalent Rect Sides", "-", "Elongation Factor", "Compactness Factor", "Heywood Circularity Factor", "Type Factor", "-", "Sum X", "Sum Y", "Sum XX", "Sum XY", "Sum YY", "Sum XXX", "Sum XXY", "Sum XYY", "Sum YYY", "-", "Moment of Inertia XX", "Moment of Inertia XY", "Moment of Inertia YY", "Moment of Inertia XXX", "Moment of Inertia XXY", "Moment of Inertia XYY", "Moment of Inertia YYY", "Norm. Moment of Inertia XX", "Norm. Moment of Inertia XY", "Norm. Moment of Inertia YY", "Norm. Moment of Inertia XXX", "Norm. Moment of Inertia XXY", "Norm. Moment of Inertia XYY", "Norm. Moment of Inertia YYY", "Hu Moment 1", "Hu Moment 2", "Hu Moment 3", "Hu Moment 4", "Hu Moment 5", "Hu Moment 6", "Hu Moment 7"]; "Rectangle"."Rotation" min=-90.0 max=90.0 step=1.0 format="%.2f"; "Rectangle"."Left" scale=0.0..1024.0; "Rectangle"."Right" scale=0.0..1024.0}
  out "CCD1 ROI参数":T29={"Rectangle big CCD1"={"Left"=1952, "Top"=1596, "Right"=570, "Bottom"=2690, "Rotation"=45.0}, "Rectangle top CCD1 "={"Left"=1952, "Top"=1596, "Right"=570, "Bottom"=2690, "Rotation"=45.0}, "Line"={"Start X"=0, "Start Y"=0, "End X"=0, "End Y"=0}, "left line "=846.0, "right line"=1152.0} {"Line"."Start X" scale=0.0..1024.0; "Line"."End X" scale=0.0..1024.0; "Rectangle top CCD1"."Rotation" format="%.2f"; "Rectangle top CCD1"."Left" scale=0.0..1024.0; "Rectangle top CCD1"."Right" scale=0.0..1024.0; "Rectangle big CCD1"."Rotation" format="%.2f"; "Rectangle big CCD1"."Left" scale=0.0..1024.0; "Rectangle big CCD1"."Right" scale=0.0..1024.0}
  out "CCD2 ROI参数":T29={"Rectangle big CCD1"={"Left"=1952, "Top"=1596, "Right"=570, "Bottom"=2690, "Rotation"=45.0}, "Rectangle top CCD1 "={"Left"=1952, "Top"=1596, "Right"=570, "Bottom"=2690, "Rotation"=45.0}, "Line"={"Start X"=0, "Start Y"=0, "End X"=0, "End Y"=0}, "left line "=846.0, "right line"=1152.0} {"Line"."Start X" scale=0.0..1024.0; "Line"."End X" scale=0.0..1024.0; "Rectangle top CCD1"."Rotation" format="%.2f"; "Rectangle top CCD1"."Left" scale=0.0..1024.0; "Rectangle top CCD1"."Right" scale=0.0..1024.0; "Rectangle big CCD1"."Rotation" format="%.2f"; "Rectangle big CCD1"."Left" scale=0.0..1024.0; "Rectangle big CCD1"."Right" scale=0.0..1024.0}
  out "CR导丝划痕检测2参数":T20={"Rectangle"={"Left"=0, "Top"=0, "Right"=0, "Bottom"=0, "Rotation"=0.0}, "Algorithm "=2, "Parameters"={"Number of Matches Requested"=1, "Minimum Match Score"=800.0, "Angle Ranges"=[{"Start Angle"=-180.0, "End Angle"=180.0}]}, "Advanced Options "=[{"Item"=102, "Value"=10.0}, {"Item"=106, "Value"=300.0}, {"Item"=107, "Value"=0.0}, {"Item"=108, "Value"=6.0}, {"Item"=109, "Value"=1.0}, {"Item"=114, "Value"=25.0}, {"Item"=111, "Value"=20.0}, {"Item"=112, "Value"=10.0}, {"Item"=113, "Value"=20.0}, {"Item"=103, "Value"=1.0}, {"Item"=104, "Value"=20.0}, {"Item"=105, "Value"=0.0}, {"Item"=100, "Value"=5.0}], "模板路径"=path "", "Color Plane "=0} {"Color Plane" items=["Red", "Green", "Blue", "Hue", "Saturation", "Luminance", "Value", "Intensity"]; "Advanced Options"."Item" items=["LD Sampling - Minimum Constrast"=0, "LD Sampling - Enable Subpixel Accuracy"=1, "LD Sampling - Search Strategy"=2, "LD Sampling - Subpixel Iterations"=3, "LD Sampling - Subpixel Tolerance"=4, "LD Sampling - Initial Match List Length"=5, "LD Sampling - Match List Reduction Factor"=6, "LD Sampling - Initial Step Size"=7, "LD Sampling - Intermediate Angular Accuracy"=8, "-"=9, "Pyramid - Max Pyramid Level"=100, "Pyramid - Minimum Contrast"=102, "Pyramid - Enable Subpixel Accuracy"=103, "Pyramid - Subpixel Iterations"=104, "Pyramid - Subpixel Tolerance"=105, "Pyramid - Initial Match List Length"=106, "Pyramid - Match List Reduction Factor"=107, "Pyramid - Intermediate Angular Accuracy"=108, "Pyramid - Process Border Matches"=109, "Pyramid - Min Match Separation Distance"=111, "Pyramid - Min Match Separation Angle"=112, "Pyramid - Max Match Overlap"=113, "Pyramid - Max Cache in MB"=114, "Pyramid - Clear Cache"=115, "-"=116, "Enable Defect Map"=200]; "Algorithm" items=["All", "Low Discrepancy Sampling", "Grayscale Value Pyramid", "Gradients Pyramid"]; "Rectangle"."Rotation" format="%.2f"; "Rectangle"."Left" scale=0.0..1024.0; "Rectangle"."Right" scale=0.0..1024.0}
  out "CR导丝划痕检测2基础参数":T9={"IsNorImage"=TRUE, "Exposure Values"=100289, "ImagePath"=path "C:/Users/hedongpo/Desktop/514-hdp/Alignment Assemble System/Test Picture/B/3.bmp"} caption="参数界面" {"Exposure Values" scale=0.0..200000.0}
  out "CR导丝缺损检测1参数":T20={"Rectangle"={"Left"=0, "Top"=0, "Right"=0, "Bottom"=0, "Rotation"=0.0}, "Algorithm "=2, "Parameters"={"Number of Matches Requested"=1, "Minimum Match Score"=800.0, "Angle Ranges"=[{"Start Angle"=-180.0, "End Angle"=180.0}]}, "Advanced Options "=[{"Item"=102, "Value"=10.0}, {"Item"=106, "Value"=300.0}, {"Item"=107, "Value"=0.0}, {"Item"=108, "Value"=6.0}, {"Item"=109, "Value"=1.0}, {"Item"=114, "Value"=25.0}, {"Item"=111, "Value"=20.0}, {"Item"=112, "Value"=10.0}, {"Item"=113, "Value"=20.0}, {"Item"=103, "Value"=1.0}, {"Item"=104, "Value"=20.0}, {"Item"=105, "Value"=0.0}, {"Item"=100, "Value"=5.0}], "模板路径"=path "", "Color Plane "=0} {"Color Plane" items=["Red", "Green", "Blue", "Hue", "Saturation", "Luminance", "Value", "Intensity"]; "Advanced Options"."Item" items=["LD Sampling - Minimum Constrast"=0, "LD Sampling - Enable Subpixel Accuracy"=1, "LD Sampling - Search Strategy"=2, "LD Sampling - Subpixel Iterations"=3, "LD Sampling - Subpixel Tolerance"=4, "LD Sampling - Initial Match List Length"=5, "LD Sampling - Match List Reduction Factor"=6, "LD Sampling - Initial Step Size"=7, "LD Sampling - Intermediate Angular Accuracy"=8, "-"=9, "Pyramid - Max Pyramid Level"=100, "Pyramid - Minimum Contrast"=102, "Pyramid - Enable Subpixel Accuracy"=103, "Pyramid - Subpixel Iterations"=104, "Pyramid - Subpixel Tolerance"=105, "Pyramid - Initial Match List Length"=106, "Pyramid - Match List Reduction Factor"=107, "Pyramid - Intermediate Angular Accuracy"=108, "Pyramid - Process Border Matches"=109, "Pyramid - Min Match Separation Distance"=111, "Pyramid - Min Match Separation Angle"=112, "Pyramid - Max Match Overlap"=113, "Pyramid - Max Cache in MB"=114, "Pyramid - Clear Cache"=115, "-"=116, "Enable Defect Map"=200]; "Algorithm" items=["All", "Low Discrepancy Sampling", "Grayscale Value Pyramid", "Gradients Pyramid"]; "Rectangle"."Rotation" format="%.2f"; "Rectangle"."Left" scale=0.0..1024.0; "Rectangle"."Right" scale=0.0..1024.0}
  out "CR导丝缺损检测1基础参数":T9={"IsNorImage"=TRUE, "Exposure Values"=100289, "ImagePath"=path "C:/Users/hedongpo/Desktop/514-hdp/Alignment Assemble System/Test Picture/B/3.bmp"} caption="参数界面" {"Exposure Values" scale=0.0..200000.0}
  out "颗粒物检测1基础参数":T14={"IsNorImage"=TRUE, "Exposure Values"=100289, "ImagePath"=path "C:/Users/hedongpo/Desktop/514-hdp/Alignment Assemble System/Test Picture/B/3.bmp", "相机选择"="cam4"} caption="参数界面" {"Exposure Values" scale=0.0..200000.0}
  in  "CR导丝划痕检测1参数":T20={"Rectangle"={"Left"=0, "Top"=0, "Right"=0, "Bottom"=0, "Rotation"=0.0}, "Algorithm "=2, "Parameters"={"Number of Matches Requested"=1, "Minimum Match Score"=800.0, "Angle Ranges"=[{"Start Angle"=-180.0, "End Angle"=180.0}]}, "Advanced Options "=[{"Item"=102, "Value"=10.0}, {"Item"=106, "Value"=300.0}, {"Item"=107, "Value"=0.0}, {"Item"=108, "Value"=6.0}, {"Item"=109, "Value"=1.0}, {"Item"=114, "Value"=25.0}, {"Item"=111, "Value"=20.0}, {"Item"=112, "Value"=10.0}, {"Item"=113, "Value"=20.0}, {"Item"=103, "Value"=1.0}, {"Item"=104, "Value"=20.0}, {"Item"=105, "Value"=0.0}, {"Item"=100, "Value"=5.0}], "模板路径"=path "", "Color Plane "=0} {"Color Plane" items=["Red", "Green", "Blue", "Hue", "Saturation", "Luminance", "Value", "Intensity"]; "Advanced Options"."Item" items=["LD Sampling - Minimum Constrast"=0, "LD Sampling - Enable Subpixel Accuracy"=1, "LD Sampling - Search Strategy"=2, "LD Sampling - Subpixel Iterations"=3, "LD Sampling - Subpixel Tolerance"=4, "LD Sampling - Initial Match List Length"=5, "LD Sampling - Match List Reduction Factor"=6, "LD Sampling - Initial Step Size"=7, "LD Sampling - Intermediate Angular Accuracy"=8, "-"=9, "Pyramid - Max Pyramid Level"=100, "Pyramid - Minimum Contrast"=102, "Pyramid - Enable Subpixel Accuracy"=103, "Pyramid - Subpixel Iterations"=104, "Pyramid - Subpixel Tolerance"=105, "Pyramid - Initial Match List Length"=106, "Pyramid - Match List Reduction Factor"=107, "Pyramid - Intermediate Angular Accuracy"=108, "Pyramid - Process Border Matches"=109, "Pyramid - Min Match Separation Distance"=111, "Pyramid - Min Match Separation Angle"=112, "Pyramid - Max Match Overlap"=113, "Pyramid - Max Cache in MB"=114, "Pyramid - Clear Cache"=115, "-"=116, "Enable Defect Map"=200]; "Algorithm" items=["All", "Low Discrepancy Sampling", "Grayscale Value Pyramid", "Gradients Pyramid"]; "Rectangle"."Rotation" format="%.2f"; "Rectangle"."Left" scale=0.0..1024.0; "Rectangle"."Right" scale=0.0..1024.0}
  out "CCD2基础参数":T9={"IsNorImage"=TRUE, "Exposure Values"=100289, "ImagePath"=path "C:/Users/hedongpo/Desktop/514-hdp/Alignment Assemble System/Test Picture/B/3.bmp"} caption="参数界面" {"Exposure Values" scale=0.0..200000.0}
  out "CCD1基础参数":T9={"IsNorImage"=TRUE, "Exposure Values"=100289, "ImagePath"=path "C:/Users/hedongpo/Desktop/514-hdp/Alignment Assemble System/Test Picture/B/3.bmp"} caption="参数界面" {"Exposure Values" scale=0.0..200000.0}
  out "CR导丝划痕检测1基础参数":T9={"IsNorImage"=TRUE, "Exposure Values"=100289, "ImagePath"=path "C:/Users/hedongpo/Desktop/514-hdp/Alignment Assemble System/Test Picture/B/3.bmp"} caption="参数界面" {"Exposure Values" scale=0.0..200000.0}
  in  "CCD2参数":T30={"Rectangle"={"Left"=1952, "Top"=146, "Right"=370, "Bottom"=2690, "Rotation"=45.0}, "Angle (degrees) "=90.0, "long"=150.0, "abgek"=-90.0, "Color"=16711680, "left threshold"=0.0, "Rectangle right"={"Left"=1952, "Top"=1596, "Right"=570, "Bottom"=2690, "Rotation"=45.0}, "long right"=150.0, "abgek right"=90.0, "Color 2"=16711680, "right threshold"=0.0, "left"=0.0, "right"=0.0, "Settings (Big)"={"Extraction Mode"=0, "Edge Threshold"=17, "Edge Filter Size"=1, "Min Length"=36, "Row Search Step Size"=13, "Col Search Step Size"=13, "Max Endpoint Gap"=10, "Closed"=FALSE, "Subpixel"=TRUE}, "Clamp Settings (Big)"={"Angle "=10.0, "Edge Polarity"={"Start"=0, "End"=0}}, " Settings top"={"Extraction Mode"=0, "Edge Threshold"=18, "Edge Filter Size"=1, "Min Length"=36, "Row Search Step Size"=64, "Col Search Step Size"=64, "Max Endpoint Gap"=10, "Closed"=FALSE, "Subpixel"=TRUE}, "Clamp Settings top "={"Angle "=10.0, "Edge Polarity"={"Start"=0, "End"=0}}, "Sub-Pixel Accuracy "=TRUE, "Threshold Parameters"={"Level Type"=enum."Absolute Value", "Threshold Level"=127, "Hysteresis"=2}, "Process "=enum."Get First + Last Edge", "Threshold Parameters 2"={"Level Type"=enum."Absolute Value", "Threshold Level"=127, "Hysteresis"=2}} {"Clamp Settings top"."Edge Polarity"."Start" items=["Any", "Rising", "Falling"]; "Clamp Settings top"."Edge Polarity"."End" items=["Any", "Rising", "Falling"]; "Settings top"."Extraction Mode" items=["Normal", "Uniform Regions"]; "Settings top"."Edge Filter Size" items=["Fine", "Normal", "Contour Tracing"]; "Settings top"."Max Endpoint Gap" min=0; "Settings top"."Col Search Step Size" min=1 max=255 step=1; "Settings top"."Row Search Step Size" min=1 max=255 step=1; "Settings top"."Min Length" min=0; "Settings top"."Edge Threshold" min=1 max=350 step=1; "Clamp Settings (Big)"."Edge Polarity"."Start" items=["Any", "Rising", "Falling"]; "Clamp Settings (Big)"."Edge Polarity"."End" items=["Any", "Rising", "Falling"]; "Settings (Big)"."Extraction Mode" items=["Normal", "Uniform Regions"]; "Settings (Big)"."Edge Filter Size" items=["Fine", "Normal", "Contour Tracing"]; "Settings (Big)"."Max Endpoint Gap" min=0; "Settings (Big)"."Col Search Step Size" min=1 max=255 step=1; "Settings (Big)"."Row Search Step Size" min=1 max=255 step=1; "Settings (Big)"."Min Length" min=0; "Settings (Big)"."Edge Threshold" min=1 max=350 step=1; "Rectangle right"."Rotation" format="%.2f"; "Rectangle right"."Left" scale=0.0..1024.0; "Rectangle right"."Right" scale=0.0..1024.0; "Rectangle"."Rotation" format="%.2f"; "Rectangle"."Left" scale=0.0..1024.0; "Rectangle"."Right" scale=0.0..1024.0}
  in  "CCD1参数":T30={"Rectangle"={"Left"=1952, "Top"=146, "Right"=370, "Bottom"=2690, "Rotation"=45.0}, "Angle (degrees) "=90.0, "long"=150.0, "abgek"=-90.0, "Color"=16711680, "left threshold"=0.0, "Rectangle right"={"Left"=1952, "Top"=1596, "Right"=570, "Bottom"=2690, "Rotation"=45.0}, "long right"=150.0, "abgek right"=90.0, "Color 2"=16711680, "right threshold"=0.0, "left"=0.0, "right"=0.0, "Settings (Big)"={"Extraction Mode"=0, "Edge Threshold"=17, "Edge Filter Size"=1, "Min Length"=36, "Row Search Step Size"=13, "Col Search Step Size"=13, "Max Endpoint Gap"=10, "Closed"=FALSE, "Subpixel"=TRUE}, "Clamp Settings (Big)"={"Angle "=10.0, "Edge Polarity"={"Start"=0, "End"=0}}, " Settings top"={"Extraction Mode"=0, "Edge Threshold"=18, "Edge Filter Size"=1, "Min Length"=36, "Row Search Step Size"=64, "Col Search Step Size"=64, "Max Endpoint Gap"=10, "Closed"=FALSE, "Subpixel"=TRUE}, "Clamp Settings top "={"Angle "=10.0, "Edge Polarity"={"Start"=0, "End"=0}}, "Sub-Pixel Accuracy "=TRUE, "Threshold Parameters"={"Level Type"=enum."Absolute Value", "Threshold Level"=127, "Hysteresis"=2}, "Process "=enum."Get First + Last Edge", "Threshold Parameters 2"={"Level Type"=enum."Absolute Value", "Threshold Level"=127, "Hysteresis"=2}} {"Clamp Settings top"."Edge Polarity"."Start" items=["Any", "Rising", "Falling"]; "Clamp Settings top"."Edge Polarity"."End" items=["Any", "Rising", "Falling"]; "Settings top"."Extraction Mode" items=["Normal", "Uniform Regions"]; "Settings top"."Edge Filter Size" items=["Fine", "Normal", "Contour Tracing"]; "Settings top"."Max Endpoint Gap" min=0; "Settings top"."Col Search Step Size" min=1 max=255 step=1; "Settings top"."Row Search Step Size" min=1 max=255 step=1; "Settings top"."Min Length" min=0; "Settings top"."Edge Threshold" min=1 max=350 step=1; "Clamp Settings (Big)"."Edge Polarity"."Start" items=["Any", "Rising", "Falling"]; "Clamp Settings (Big)"."Edge Polarity"."End" items=["Any", "Rising", "Falling"]; "Settings (Big)"."Extraction Mode" items=["Normal", "Uniform Regions"]; "Settings (Big)"."Edge Filter Size" items=["Fine", "Normal", "Contour Tracing"]; "Settings (Big)"."Max Endpoint Gap" min=0; "Settings (Big)"."Col Search Step Size" min=1 max=255 step=1; "Settings (Big)"."Row Search Step Size" min=1 max=255 step=1; "Settings (Big)"."Min Length" min=0; "Settings (Big)"."Edge Threshold" min=1 max=350 step=1; "Rectangle right"."Rotation" format="%.2f"; "Rectangle right"."Left" scale=0.0..1024.0; "Rectangle right"."Right" scale=0.0..1024.0; "Rectangle"."Rotation" format="%.2f"; "Rectangle"."Left" scale=0.0..1024.0; "Rectangle"."Right" scale=0.0..1024.0}
  # "E:\\Labview项目\\Steering Wheel AOI System\\Source Code"
  # "Range"
  # "C:\\Users\\delluser001\\Desktop\\铜垫片检测\\LX Inspect System\\Source Code"
  # "active 0:高电平变为低电平时，产生急停信号\nactive 1:低电平变为高电平时，产生急停信号"
  # "箭头指示参数"
  # "箭头指示参数"
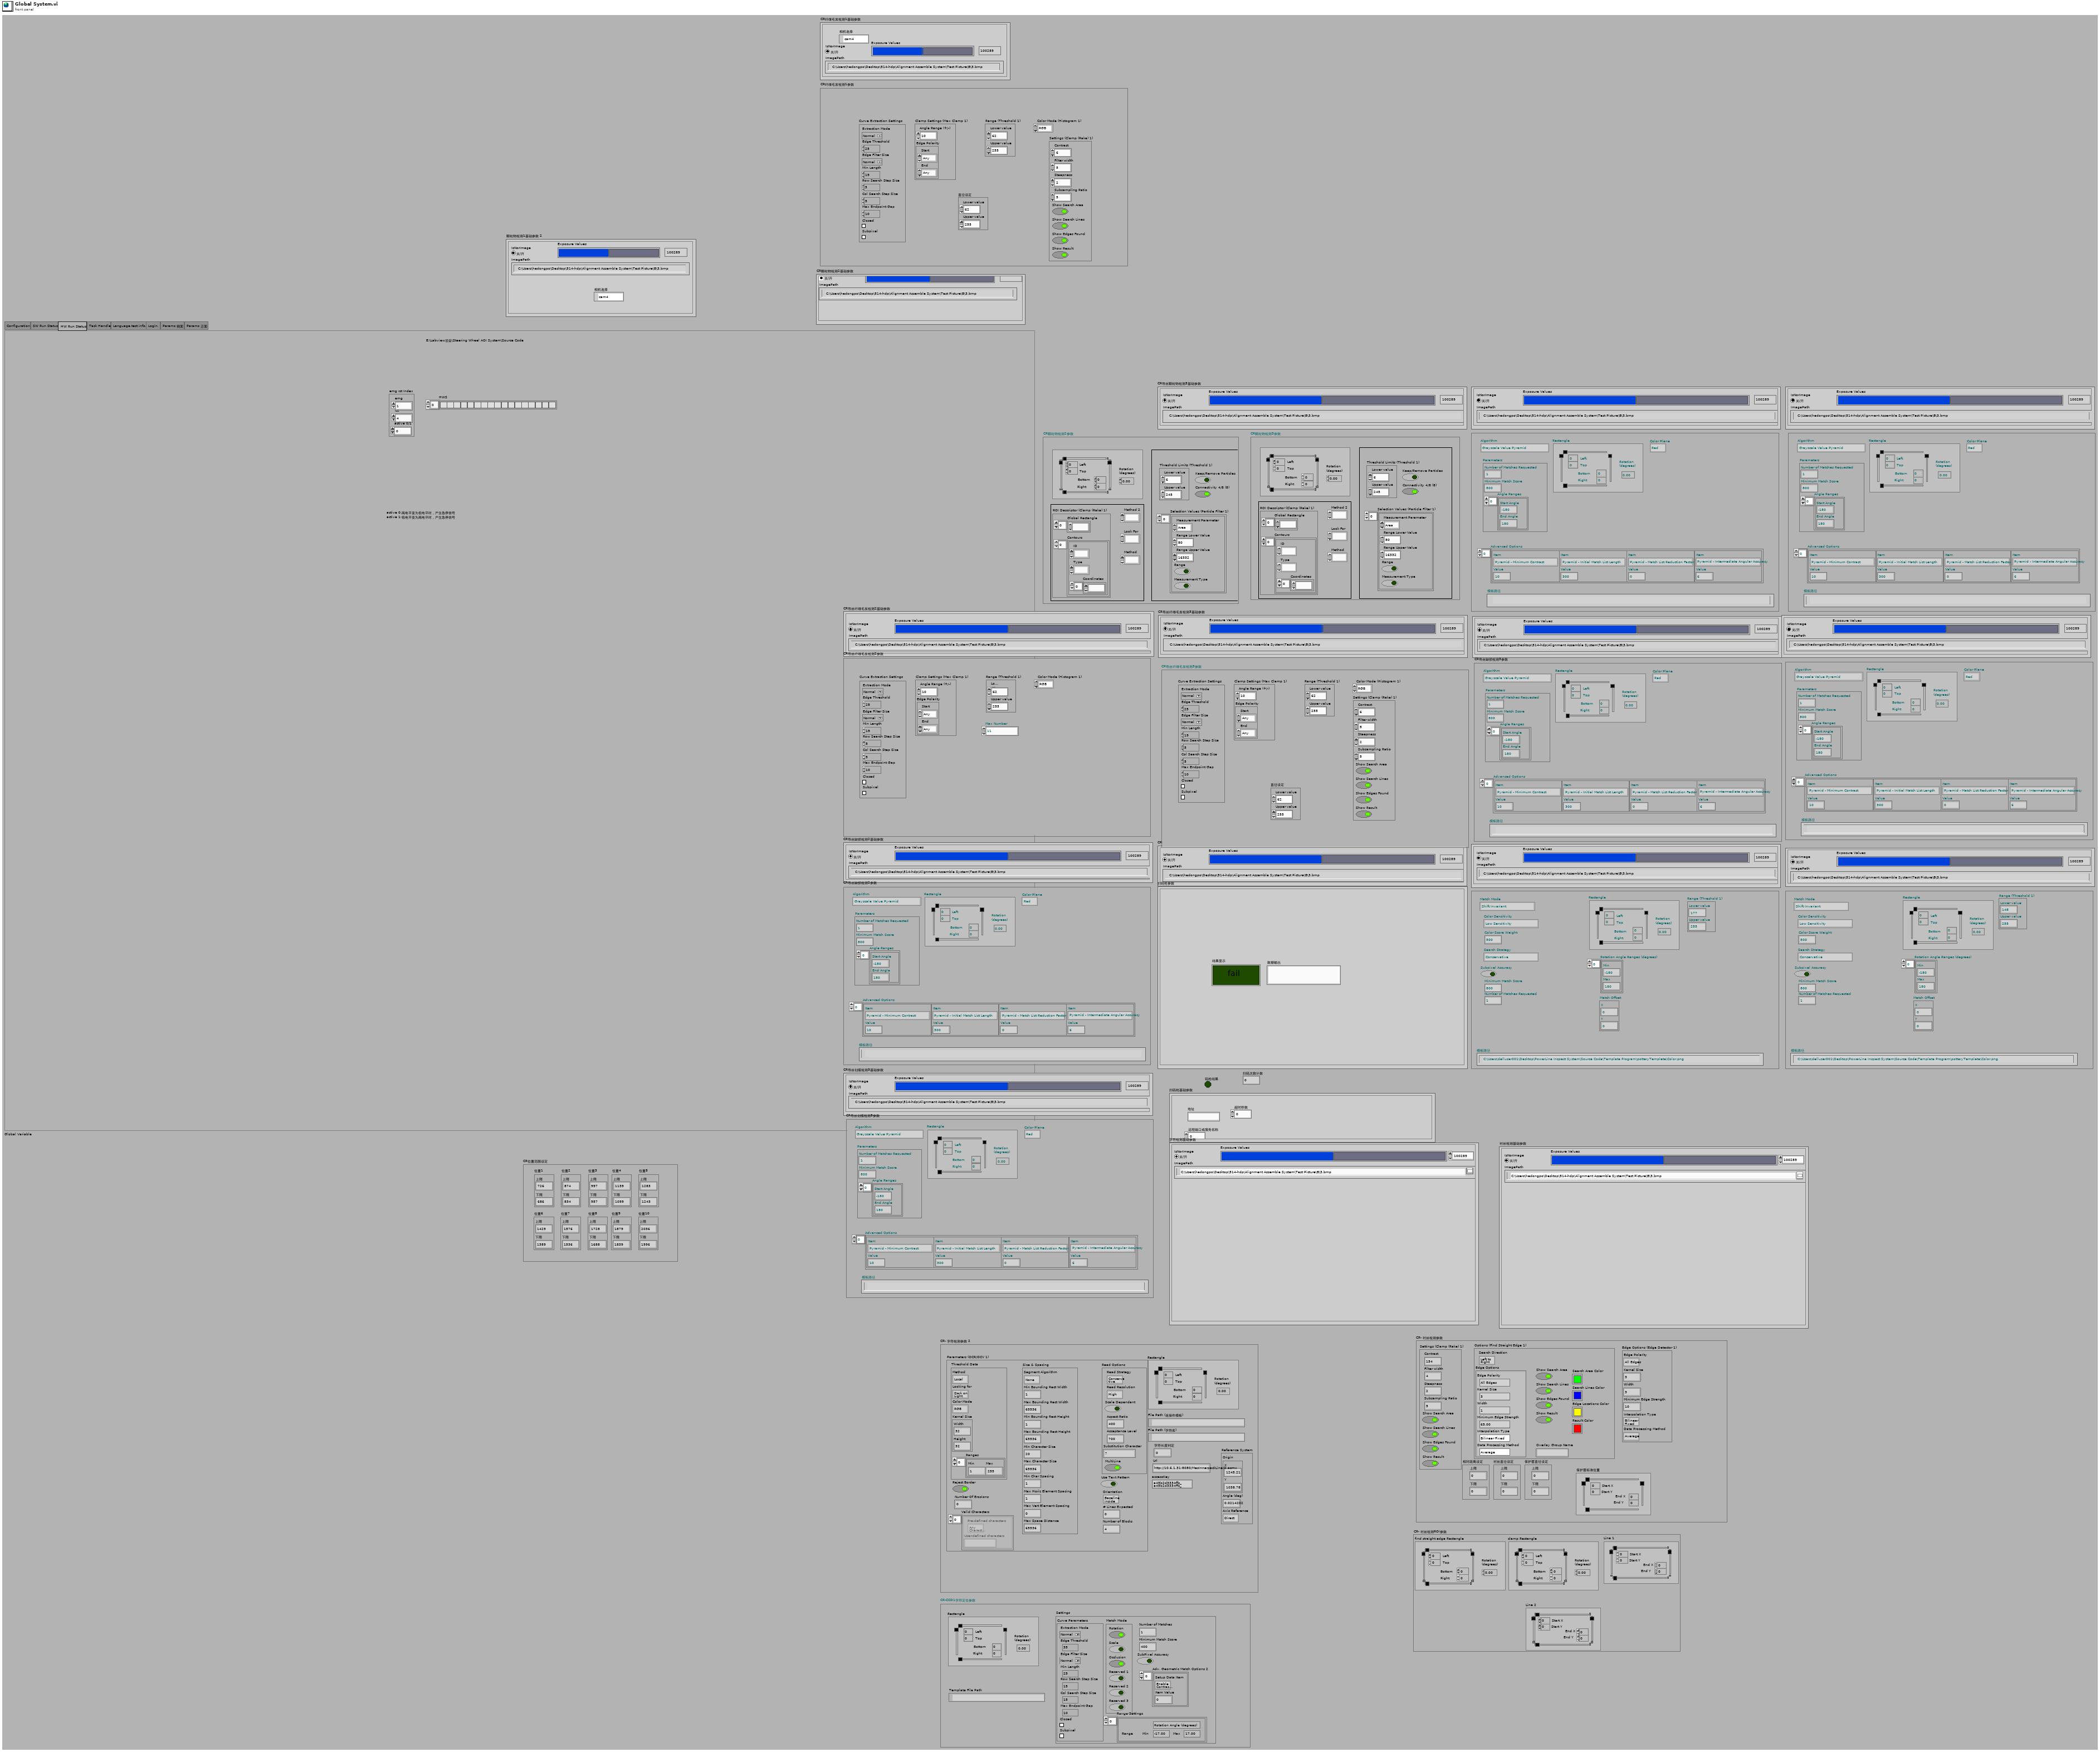
[diagram p1: front panel]
types:
  T1 = typedef "IMAQ Rectangle" = cluster{"Left":i32, "Top":i32, "Right":i32, "Bottom":i32, "Rotation":dbl}
  T2 = typedef "IMAQ Curve Parameters.ctl" = cluster{"Extraction Mode":u32, "Edge Threshold":i32, "Edge Filter Size":u32, "Min Length":i32, "Row Search Step Size":i32, "Col Search Step Size":i32, "Max Endpoint Gap":i32, "Closed":bool, "Subpixel":bool}
  T3 = typedef "IMAQ Match Range Setting.ctl" = cluster{"Match Constraints":u32, "Min":dbl, "Max":dbl}
  T4 = cluster{"Rectangle":T1, "Settings":cluster{"Curve Parameters":T2, "Match Mode":cluster{"Rotation":bool, "Scale":bool, "Occlusion":bool, "Reserved 1":bool, "Reserved 2":bool, "Reserved 3":bool}, "Range Settings":T3[], "Number of Matches":i32, "Minimum Match Score":sgl, "SubPixel Accuracy":bool, "Adv. Geometric Match Options 2":cluster{"Setup Data Item":u16, "Item Value":dbl}[]}, "Template File Path":path}
  T5 = cluster{"位置1":cluster{"上限":dbl, "下限":dbl}, "位置2":cluster{"上限":dbl, "下限":dbl}, "位置3":cluster{"上限":dbl, "下限":dbl}, "位置4":cluster{"上限":dbl, "下限":dbl}, "位置5":cluster{"上限":dbl, "下限":dbl}, "位置6":cluster{"上限":dbl, "下限":dbl}, "位置7":cluster{"上限":dbl, "下限":dbl}, "位置8":cluster{"上限":dbl, "下限":dbl}, "位置9":cluster{"上限":dbl, "下限":dbl}, "位置10":cluster{"上限":dbl, "下限":dbl}}
  T6 = cluster{"Parameters (OCR/OCV 1)":cluster{"Threshold Data":cluster{"Method":enum16{"Fixed Range", "Uniform", "Linear", "Non Linear", "Local", "Color"}, "Looking for":u32, "Color Mode":u32, "Kernel Size":cluster{"Width":i32, "Height":i32}, "Ranges":cluster{"Min":i32, "Max":i32}[]}, "Reject Border":bool, "Number Of Erosions":i32, "Size & Spacing":cluster{"Segment Algorithm":u16, "Min Bounding Rect Width":i32, "Max Bounding Rect Width":i32, "Min Bounding Rect Height":i32, "Max Bounding Rect Height":i32, "Min Character Size":i32, "Max Character Size":i32, "Min Char Spacing":i32, "Max Horiz Element Spacing":i32, "Max Vert Element Spacing":i32, "Max Space Distance":i32}, "Read Options":cluster{"Read Strategy":i32, "Read Resolution":i32, "Scale Dependant":bool, "Aspect Ratio":i32, "Acceptance Level":i32, "Substitution Character":string, "MultiLine":bool}, "Valid Characters":cluster{"Pre-defined characters":i32, "User-defined characters":string}[], "Use Text Pattern":bool, "Orientation":u32, "# Lines Expected":u32, "Number of Blocks":i32}, "Rectangle":T1, "字符长度判定":dbl, "Reference System":cluster{"Origin":cluster{"X":sgl, "Y":sgl}, "Angle (deg)":sgl, "Axis Reference":u32}, "File Path (字符库)":path, "File Path (连接件模板)":path, "Url":string, "accessKey":string}
  T7 = typedef "IMAQ Line" = cluster{"Start X":i32, "Start Y":i32, "End X":i32, "End Y":i32}
  T8 = cluster{"find straight edge Rectangle":T1, "Line 1":T7, "clamp Rectangle ":T1, "Line 2":T7}
  T9 = cluster{"IsNorImage":bool, "Exposure Values":u32, "ImagePath":path}
  T10 = typedef "Edge Options.ctl" = cluster{"Edge Polarity":T11, "Kernel Size":u32, "Width":u32, "Minimum Edge Strength":sgl, "Interpolation Type":enum32{"Zero Order", "Bilinear", "Quadratic", "Cubic", "Bilinear Fixed"}, "Data Processing Method":enum32{"Average", "Median"}}
  T11 = typedef "Edge Polarity.ctl" = u32
  T12 = cluster{"Settings (Clamp (Rake) 1)":cluster{"Contrast":i32, "Filter width":i32, "Steepness":i32, "Subsampling Ratio":u32, "Show Search Area":bool, "Show Search Lines":bool, "Show Edges Found":bool, "Show Result":bool}, "Options (Find Straight Edge 1)":cluster{"Search Direction":u32, "Edge Options":T10, "Show Search Area":bool, "Show Search Lines":bool, "Show Edges Found":bool, "Show Result":bool, "Search Area Color":u32, "Search Lines Color":u32, "Edge Locations Color":u32, "Result Color":u32, "Overlay Group Name":string}, "相对距离设定":cluster{"上限":dbl, "下限":dbl}, "衬丝直径设定":cluster{"上限":dbl, "下限":dbl}, "保护套直径设定":cluster{"上限":dbl, "下限":dbl}, "Edge Options (Edge Detector 1)":cluster{"Edge Polarity":u32, "Kernel Size":u32, "Width":u32, "Minimum Edge Strength":sgl, "Interpolation Type":enum32{"Zero Order", "Bilinear", "Quadratic", "Cubic", "Bilinear Fixed"}, "Data Processing Method":enum32{"Average", "Median"}}, "保护套标准位置":T7}
  T13 = typedef "IMAQdx.ctl" = refnum<k21>
  T14 = cluster{"IsNorImage":bool, "Exposure Values":u32, "ImagePath":path, "相机选择":T13}
  T15 = cluster{"地址":string, "远程端口或服务名称":u16, "超时秒数":dbl}
  T16 = cluster{"Curve Extraction Settings ":T2, "Color Mode (Histogram 1)":u16, "Range (Threshold 1)":cluster{"Lower value":sgl, "Upper value":sgl}, "Clamp Settings (Max Clamp 1)":cluster{"Angle Range (+/-)":dbl, "Edge Polarity":cluster{"Start":u32, "End":u32}}, "Settings (Clamp (Rake) 1)":cluster{"Contrast":i32, "Filter width":i32, "Steepness":i32, "Subsampling Ratio":u32, "Show Search Area":bool, "Show Search Lines":bool, "Show Edges Found":bool, "Show Result":bool}, "直径设定":cluster{"Lower value":sgl, "Upper value":sgl}}
  T17 = cluster{"Rectangle":T1, "Threshold Limits (Threshold 1)":cluster{"Lower value":sgl, "Upper value":sgl}, "Keep/Remove Particles ":bool, "Connectivity 4/8 (8) ":bool, "Selection Values (Particle Filter 1)":cluster{"Measurement Parameter":i32, "Range Lower Value":dbl, "Range Upper Value":dbl, "Range":bool, "Measurement Type":bool}[], "Corner Options (Feature Detection 1)":cluster{"Detector type":enum32{"Harris Corner", "Shi-Tomasi Corner"}, "Kernel size":i32, "Min Corner Point Strength":dbl}, "Pyramid level (Feature Detection 1)":u32, "Method ":i32, "Look For":u32, "Method 2":i32, "ROI Descriptor (Clamp (Rake) 1)":cluster{"Global Rectangle":i32[], "Contours":cluster{"ID":enum32{"External", "Internal"}, "Type":u32, "Coordinates":i32[]}[]}}
  T18 = cluster{"IsNorImage":bool, "Exposure Values":u32, "ImagePath":path, "数据输出":string, "结果显示":bool}
  T19 = cluster{"Rectangle":T1, "模板路径":path, "Match Mode ":u32, "Minimum Match Score ":sgl, "Number of Matches Requested":i32, "Rotation Angle Ranges (degrees)":cluster{"Min":sgl, "Max":sgl}[], "Color Sensitivity ":u32, "Match Offset":cluster{"X":sgl, "Y":sgl}, "Color Score Weight ":sgl, "Search Strategy ":u32, "Subpixel Accuracy ":bool, "Range (Threshold 1)":cluster{"Lower value":sgl, "Upper value":sgl}}
  T20 = cluster{"Rectangle":T1, "Algorithm ":i32, "Parameters":cluster{"Number of Matches Requested":i32, "Minimum Match Score":sgl, "Angle Ranges":cluster{"Start Angle":sgl, "End Angle":sgl}[]}, "Advanced Options ":cluster{"Item":u16, "Value":dbl}[], "模板路径":path, "Color Plane ":i32}
  T21 = cluster{"Max Number":sgl, "Curve Extraction Settings ":T2, "Color Mode (Histogram 1)":u16, "Range (Threshold 1)":cluster{"Lower value":sgl, "Upper value":sgl}, "Clamp Settings (Max Clamp 1)":cluster{"Angle Range (+/-)":dbl, "Edge Polarity":cluster{"Start":u32, "End":u32}}}
  T22 = enum32{"Configuration", "SW Run Status", "HW Run Status", "Task Handle", "Language,test info,", "Login,", "Params 侧面", "Params 正面"}
  T23 = typedef "IMAQ Image.ctl" = refnum<image>
  T24 = cluster{"case name":string[], "queue array":refnum<queue>[]}
  T25 = cluster{"UserName":string, "LoginTime":string, "level":string, "UserGroup":string}
  T26 = typedef "Straight Edge Options.ctl" = cluster{"Number of Lines":i32, "Type":T27, "Min. Score":dbl, "Max. Score":dbl, "Orientation":dbl, "Angle Range":dbl, "Angle Tolerance":dbl, "Step Size":u32, "Min. SNR (db)":dbl, "Min. Points (%)":dbl, "Hough Iterations":i32}
  T27 = typedef "Straight Edge Process.ctl" = enum32{"First Edge Rake", "Best Edge Rake", "Hough Edge Rake", "First Edge Projection", "Best Edge Projection"}
  T28 = cluster{"Rectangle":T1, "Find Straight Edge 1":T26, "Process (Edge Detector 1)":enum16{"Get First Edge", "Get First + Last Edge", "Get All Edges", "Get Best Edge"}, "Edge Options (Edge Detector 1)":cluster{"Edge Polarity":u32, "Kernel Size":u32, "Width":u32, "Minimum Edge Strength":sgl, "Interpolation Type":enum32{"Zero Order", "Bilinear", "Quadratic", "Cubic", "Bilinear Fixed"}, "Data Processing Method":enum32{"Average", "Median"}}, "Options (Find Straight Edge 1)":cluster{"Search Direction":u32, "Edge Options":T10, "Show Search Area":bool, "Show Search Lines":bool, "Show Edges Found":bool, "Show Result":bool, "Search Area Color":u32, "Search Lines Color":u32, "Edge Locations Color":u32, "Result Color":u32, "Overlay Group Name":string}, "Parameters (Pattern Matching 1)":cluster{"Number of Matches Requested":i32, "Minimum Match Score":sgl, "Angle Ranges":cluster{"Start Angle":sgl, "End Angle":sgl}[]}, "Template File Path (Pattern Matching 1)":path}
  T29 = cluster{"Rectangle big CCD1":T1, "Rectangle top CCD1 ":T1, "Line":T7, "left line ":dbl, "right line":dbl}
  T30 = cluster{"Rectangle":T1, "Angle (degrees) ":sgl, "long":sgl, "abgek":dbl, "Color":u32, "left threshold":dbl, "Rectangle right":T1, "long right":sgl, "abgek right":dbl, "Color 2":u32, "right threshold":dbl, "left":dbl, "right":dbl, "Settings (Big)":T2, "Clamp Settings (Big)":cluster{"Angle ":dbl, "Edge Polarity":cluster{"Start":u32, "End":u32}}, " Settings top":T2, "Clamp Settings top ":cluster{"Angle ":dbl, "Edge Polarity":cluster{"Start":u32, "End":u32}}, "Sub-Pixel Accuracy ":bool, "Threshold Parameters":cluster{"Level Type":enum32{"Absolute Value", "Relative value"}, "Threshold Level":i32, "Hysteresis":i32}, "Process ":enum16{"Get First Edge", "Get First + Last Edge", "Get All Edges"}, "Threshold Parameters 2":cluster{"Level Type":enum32{"Absolute Value", "Relative value"}, "Threshold Level":i32, "Hysteresis":i32}}
diagram:
